vi "Example - Fading (Basic).vi"() -> ()   [LabVIEW 2012]
doc: "This example shows how to use the UI Tools Fade In & Out primitives to play with transparency when dealing with dialog boxes or interrface loading."
uses:
  _Commands_Example.ctl
  Fading/_Fade In(I32).vi
  Fading/_Fade Out(I32).vi
panel:
  in  "About":bool caption="Press this button to simulate a dialog box call."
  in  "Exit":bool caption="Exits with a fade out"
  # "Press the ? button to call up a Dialog Box with Fade in & out.\nPress Exit to Fade out and quit."
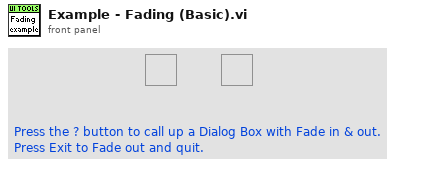
[diagram p1: front panel]
types:
  T1 = typedef "_Commands_Example.ctl" = enum16{"Idle", "Init", "OpenFP", "CloseFP", "Fade - Partial", "About", "Exit"}
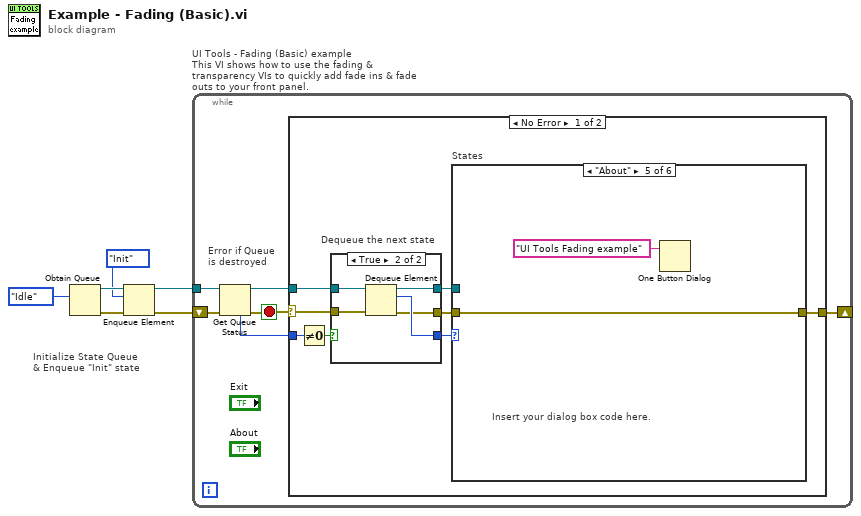
[diagram p0: block diagram]
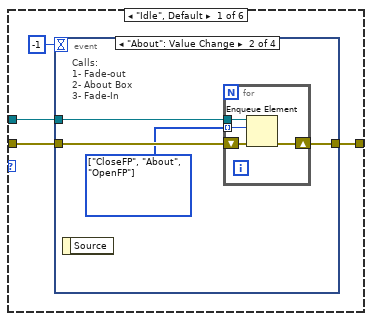
[diagram p2: hidden frame]
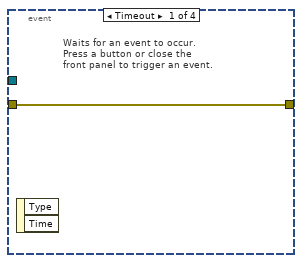
[diagram p3: hidden frame]
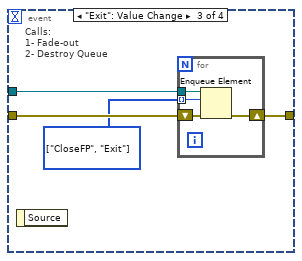
[diagram p4: hidden frame]
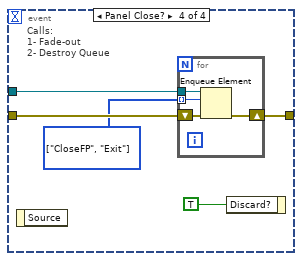
[diagram p5: hidden frame]
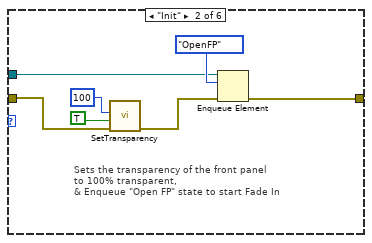
[diagram p6: hidden frame]
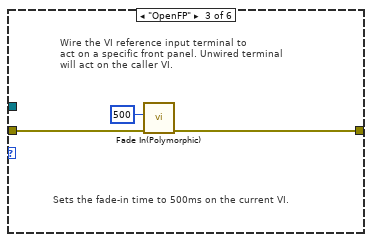
[diagram p7: hidden frame]
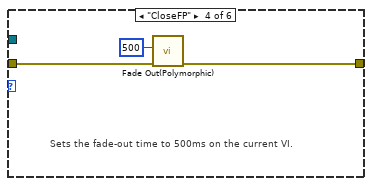
[diagram p8: hidden frame]
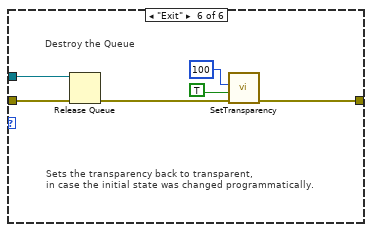
[diagram p9: hidden frame]
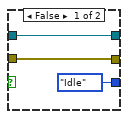
[diagram p10: hidden frame]
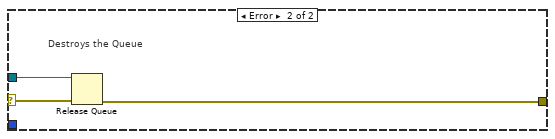
[diagram p11: hidden frame]
diagram:
  # "Initialize State Queue\n& Enqueue \"Init\" state"
  n1 = Obtain Queue(element data type=_Commands_Example."Idle" ("Commands")) -> (queue out=w6:refnum<queue>, error out=w4:errorcluster)  [unwired: 3 in, 2 out]
  n2 = Enqueue Element(queue=w6, element=_Commands_Example."Init" ("Commands"), error in (no error)=w4) -> (queue out=w2:refnum<queue>, error out=w3:errorcluster)  [unwired: 2 out]
  n3 = while "UI Tools - Fading (Basic) example\nThis VI shows how to use the fading & transparency VIs to quickly add fade ins & fade outs to your front panel." {
    tunnel: w2 -> [w11]
    shift-right: [w7] -> _
    shift-left: w3 -> [w12]
    stop <- w9 stop-if-true
    # "Error if Queue\nis destroyed"
    n4 = Get Queue Status(queue=w11, error in (no error)=w12) -> (queue out=w8:refnum<queue>, error out=w9:errorcluster, # elements in queue=w10:i32)  [unwired: 6 out]
    n5 = case shown="No Error" w9 {
      selector: w9 -> [w17 w81]
      tunnel: w10 -> [w20 _]
      tunnel: w8 -> [w18 w82]
      tunnel: [w13 w80] -> w7
      frame No Error {
        # "Dequeue the next state"
        n6 = Not Equal To 0?(x=w20) -> (x != 0?=w19:bool)
        n7 = case shown="True" w19 {
          tunnel: w18 -> [w74 w79]
          tunnel: w17 -> [w73 w78]
          tunnel: [_Commands_Example."Idle" ("Commands") w77] -> w16
          tunnel: [w74 w76] -> w15
          tunnel: [w73 w75] -> w14
          frame False {
          }
          frame True {
            n8 = Dequeue Element(queue=w79, error in (no error)=w78) -> (queue out=w76:refnum<queue>, element=w77:T1, error out=w75:errorcluster)  [unwired: 2 out]
          }
        }
        n9 = case "States" shown="\"About\"" w16 {
          tunnel: w15 -> [w23 w56 _ _ _ w70]
          tunnel: w14 -> [w22 w52 w59 w62 w65 w71]
          tunnel: [w21 w51 w58 w61 w65 w66] -> w13
          frame "Idle", Default {
            n10 = event shown="[1] \"About\": Value Change" {
              selector: _ -> [_ _ _ _]
              dyn-events: _ -> [_ _ _ _]
              timeout: -1 -> [_ _ _ _]
              tunnel: w23 -> [_ w29 w37 w46]
              tunnel: w22 -> [w25 w28 w36 w45]
              tunnel: [w25 w26 w34 w43] -> w21
              event Timeout {
                # "Waits for an event to occur.\nPress a button or close the\nfront panel to trigger an event."
                n11 = event-data() -> ()  [unwired: 3 out]
              }
              event "About": Value Change {
                w27 = T1[] [enum."CloseFP", enum."About", enum."OpenFP"] items=["Idle", "Init", "OpenFP", "CloseFP", "Fade - Partial", "About", "Exit"]
                # "Calls: \n1- Fade-out\n2- About Box\n3- Fade-In"
                n12 = event-data() -> ()  [unwired: 2 out]
                n13 = for {
                  tunnel: w29 -> [w33]
                  tunnel: w27 -> [w31] mode=indexing
                  shift-right: [w30] -> w26
                  shift-left: w28 -> [w32]
                  n14 = Enqueue Element(queue=w33, element=w31, error in (no error)=w32) -> (error out=w30:errorcluster)  [unwired: 3 out]
                }
              }
              event "Exit": Value Change {
                w35 = T1[] [enum."CloseFP", enum."Exit"] items=["Idle", "Init", "OpenFP", "CloseFP", "Fade - Partial", "About", "Exit"]
                # "Calls: \n1- Fade-out\n2- Destroy Queue"
                n15 = event-data() -> ()  [unwired: 2 out]
                n16 = for {
                  tunnel: w37 -> [w41]
                  tunnel: w35 -> [w39] mode=indexing
                  shift-right: [w38] -> w34
                  shift-left: w36 -> [w40]
                  n17 = Enqueue Element(queue=w41, element=w39, error in (no error)=w40) -> (error out=w38:errorcluster)  [unwired: 3 out]
                }
              }
              event Panel Close? {
                w44 = T1[] [enum."CloseFP", enum."Exit"] items=["Idle", "Init", "OpenFP", "CloseFP", "Fade - Partial", "About", "Exit"]
                # "Calls: \n1- Fade-out\n2- Destroy Queue"
                n18 = event-data() -> ()  [unwired: 2 out]
                n19 = for {
                  tunnel: w46 -> [w50]
                  tunnel: w44 -> [w48] mode=indexing
                  shift-right: [w47] -> w43
                  shift-left: w45 -> [w49]
                  n20 = Enqueue Element(queue=w50, element=w48, error in (no error)=w49) -> (error out=w47:errorcluster)  [unwired: 3 out]
                }
                n21 = event-data("Discard?"=TRUE) -> ()  [unwired: 1 in, 1 out]
              }
            }
          }
          frame "Init" {
            # "Sets the transparency of the front panel\nto 100% transparent,\n& Enqueue \"Open FP\" state to start Fade In"
            n22 = call "SetTransparency.vi"("error in"=w52, "Run VI Transparently (T)"=TRUE, "Transparency (%)"=100) -> ("error out"=w53:errorcluster)  [unwired: 1 in, 7 out]
            n23 = Enqueue Element(queue=w56, element=_Commands_Example."OpenFP" ("Commands"), error in (no error)=w53) -> (error out=w51:errorcluster)  [unwired: 3 out]
          }
          frame "OpenFP" {
            # "Wire the VI reference input terminal to\nact on a specific front panel. Unwired terminal\nwill act on the caller VI."
            # "Sets the fade-in time to 500ms on the current VI."
            n24 = call-poly "Fade In(Polymorphic).vi"("error in"=w59, "Fade time (ms)"=500) -> ("error out"=w58:errorcluster)  [unwired: 2 in, 7 out]
          }
          frame "CloseFP" {
            # "Sets the fade-out time to 500ms on the current VI."
            n25 = call-poly "Fade Out(Polymorphic).vi"("error in"=w62, "Fade time (ms)"=500) -> ("error out"=w61:errorcluster)  [unwired: 2 in, 7 out]
          }
          frame "About" {
            # "Insert your dialog box code here."
            n26 = One Button Dialog(message="UI Tools Fading example") -> ()  [unwired: 2 out]
          }
          frame "Exit" {
            # "Destroy the Queue"
            # "Sets the transparency back to transparent, \nin case the initial state was changed programmatically."
            n27 = Release Queue(queue=w70, error in (no error)=w71) -> (error out=w67:errorcluster)  [unwired: 3 out]
            n28 = call "SetTransparency.vi"("error in"=w67, "Run VI Transparently (T)"=TRUE, "Transparency (%)"=100) -> ("error out"=w66:errorcluster)  [unwired: 1 in, 7 out]
          }
        }
      }
      frame Error {
        # "Destroys the Queue"
        n29 = Release Queue(queue=w82, error in (no error)=w81) -> (error out=w80:errorcluster)  [unwired: 3 out]
      }
    }
  }
